vi "HEWH RLT Update Panel Information.vi"(0 "Station D In":T1, 1 "Station C In":T1, 2 "Station B In":T1, 3 "Station A In":T1, 5 "Error In":errorcluster, 8 "Panel":T3[][](array[typedef]), 9 "MW 100 Channel Input":string[](array[string])) -> (14 "Station D Out":T1, 15 "Station C Out":T1, 16 "Station B Out":T1, 17 "Station A Out":T1, 19 "Error Out":errorcluster)   [LabVIEW 2016]
uses:
  Type Definitions/HEWH RLT Stations.ctl
  Type Definitions/HEWH Label Channel.ctl
  Type Definitions/HEWH Channel Label RLT.ctl
  Custom Instrument Control/MW100/Type Definitions/Station ID Selector.ctl
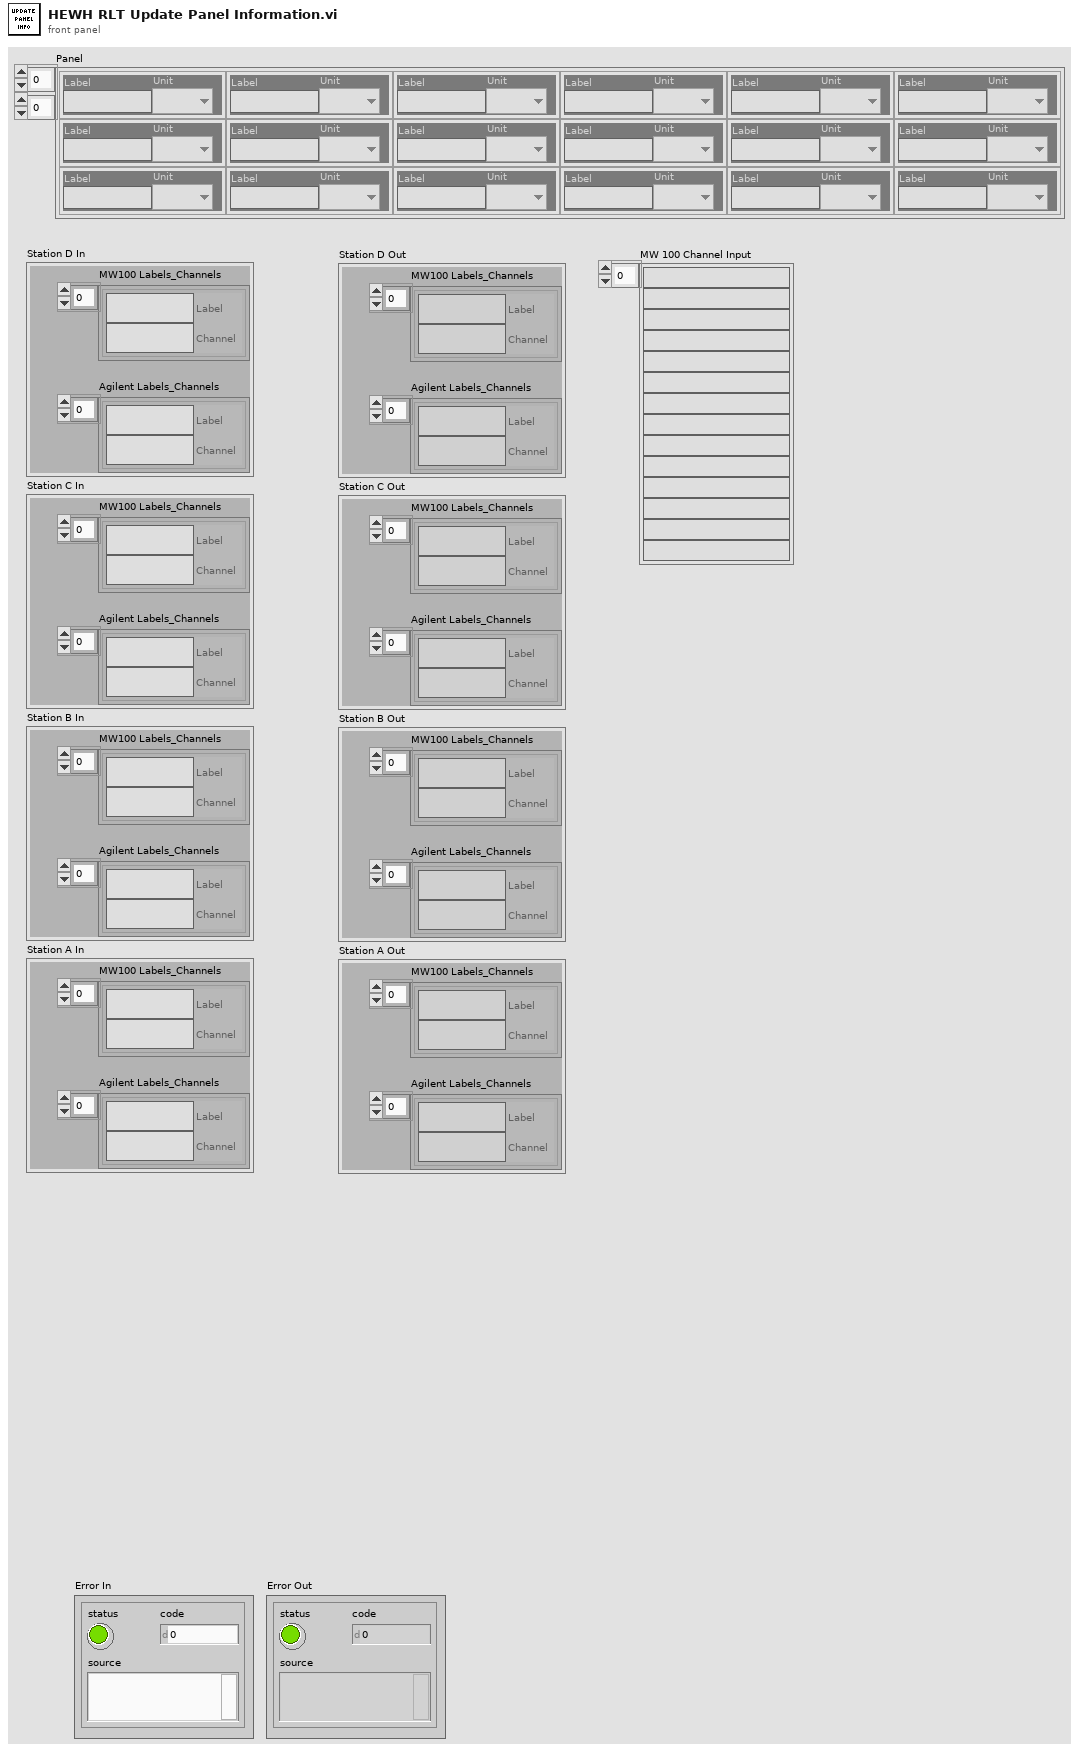
[diagram p1: front panel]
types:
  T1 = typedef "HEWH RLT Stations.ctl" = cluster{"MW100 Labels_Channels":T2[], "Agilent Labels_Channels":T2[]}
  T2 = typedef "HEWH Label Channel.ctl" = cluster{"Label":string, "Channel":string}
  T3 = typedef "HEWH Channel Label RLT.ctl" = cluster{"Label":string, "Unit":T4}
  T4 = typedef "Station ID Selector.ctl" = enum16{"", "A", "B", "C", "D", "Global"}
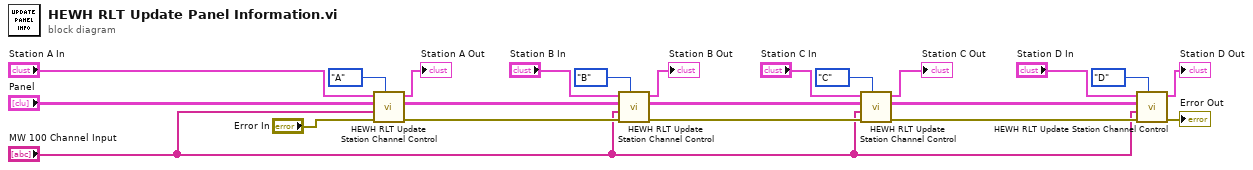
[diagram p0: block diagram]
diagram:
  n1 = call "HEWH RLT Update Station Channel Control.vi"("Unit"=Station_ID_Selector."A", "Error In"="Error In", "TC Channels"="MW 100 Channel Input", "Panel In"="Panel", "Station In"="Station A In") -> ("Error Out"=w16:errorcluster, "Panel Out"=w12:T3[][], "Station Out"=→"Station A Out":T1)  [unwired: 4 in]
  n2 = call "HEWH RLT Update Station Channel Control.vi"("Unit"=Station_ID_Selector."B", "Error In"=w16, "TC Channels"="MW 100 Channel Input", "Panel In"=w12, "Station In"="Station B In") -> ("Error Out"=w11:errorcluster, "Panel Out"=w8:T3[][], "Station Out"=→"Station B Out":T1)  [unwired: 4 in]
  n3 = call "HEWH RLT Update Station Channel Control.vi"("Unit"=Station_ID_Selector."C", "Error In"=w11, "TC Channels"="MW 100 Channel Input", "Panel In"=w8, "Station In"="Station C In") -> ("Error Out"=w7:errorcluster, "Panel Out"=w6:T3[][], "Station Out"=→"Station C Out":T1)  [unwired: 4 in]
  n4 = call "HEWH RLT Update Station Channel Control.vi"("Unit"=Station_ID_Selector."D", "Error In"=w7, "TC Channels"="MW 100 Channel Input", "Panel In"=w6, "Station In"="Station D In") -> ("Error Out"=→"Error Out":errorcluster, "Station Out"=→"Station D Out":T1)  [unwired: 4 in, 1 out]
